vi "Append to Array - String.vi"(0 "JSON Tree in (JSON Array)":variant, 5 "String":string, 11 "error in (no error)":errorcluster) -> (4 "JSON Tree out (JSON Array)":variant, 15 "error out":errorcluster)   [LabVIEW 2015, in "i3-json.lvlib"]
doc: "Use this template to build a VI to use as a subVI."
uses:
  i3-json.lvlib
  JSON Types/JSON Type.ctl
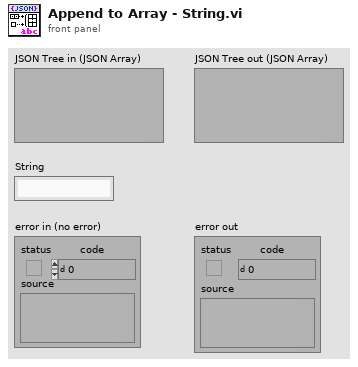
[diagram p1: front panel]
types:
  T1 = typedef "i3-json.lvlib/JSON Type.ctl" = enum8{"JSON Compatible", "JSON Array", "JSON Object", "JSON Null", "Double", "String", "Boolean", "Unknown"}
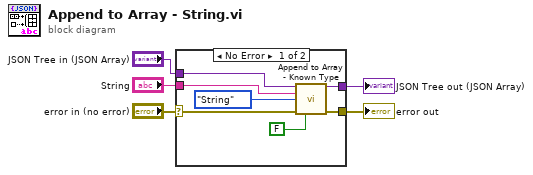
[diagram p0: block diagram]
diagram:
  n1 = case shown="No Error" "error in (no error)" {
    selector: "error in (no error)" -> [w10 w14]
    tunnel: [w11 w14] -> w4
    tunnel: [w12 w13] -> w3
    tunnel: "JSON Tree in (JSON Array)" -> [w9 w13]
    tunnel: "String" -> [w8 _]
    frame No Error {
      n2 = call "Append to Array - Known Type.vi"("JSON Tree in (JSON Array)"=w9, "Value"=w8, "JSON Type"=JSON_Type."String", "error in (no error)"=w10, "Add Parameter as JSON Tree?"=FALSE) -> ("JSON Tree out (JSON Array)"=w12:variant, "error out"=w11:errorcluster)  [unwired: 9 in]
    }
    frame Error {
    }
  }
  "error out" <- w4
  "JSON Tree out (JSON Array)" <- w3
